vi "cblas zherk.vi"(0 "A":T4, 2 "C":T4, 3 "alpha":dbl=1.0, 4 "beta":dbl=1.0, 5 "order":T3=101 items=["CblasRowMajor"=101, "CblasColMajor"=102], 6 "transA":T1=111 items=["CblasNoTrans"=111, "CblasTrans"=112, "CblasConjTrans "=113], 7 "uplo":T2=121 items=["CblasUpper"=121, "CblasLower"=122], 8 "lda":i32, 11 "n":i32=-1, 12 "ldc":i32, 13 "k":i32=-1) -> (14 "zherk":T4, 19 "error":i32)   [LabVIEW 2017, in "NI_AALBLAS.lvlib"]
uses:
  NI_AALBLAS.lvlib
  ComplexMatrix.ctl
  Order.ctl
  UpLo.ctl
  Operation_Transpose.ctl
  NI_Matrix.lvlib
  lvblas.dll
panel:
  # "void cblas_zherk(order, uplo, transA, n, k, alpha,*A, lda, beta, *C, ldc)"
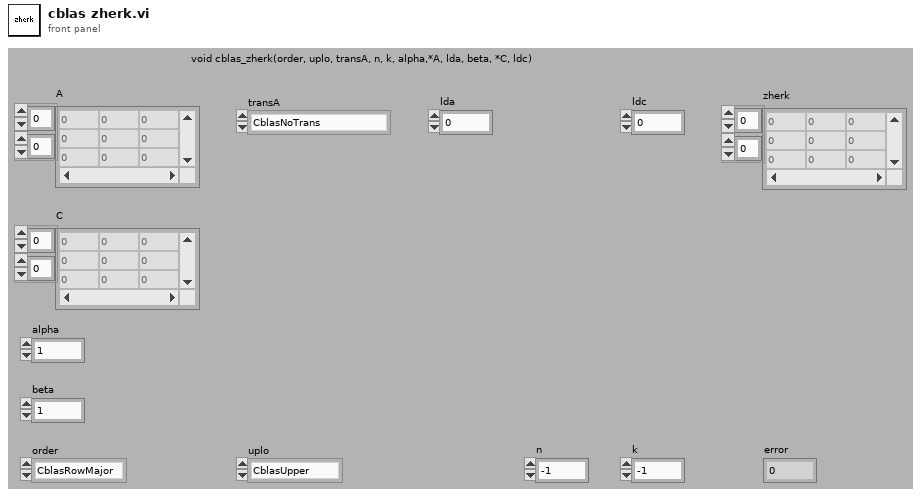
[diagram p1: front panel]
types:
  T1 = typedef "NI_AALBLAS.lvlib/Operation_Transpose.ctl" = i32
  T2 = typedef "NI_AALBLAS.lvlib/UpLo.ctl" = i32
  T3 = typedef "NI_AALBLAS.lvlib/Order.ctl" = i32
  T4 = typedef "NI_Matrix.lvlib/ComplexMatrix.ctl" = cdb[][]
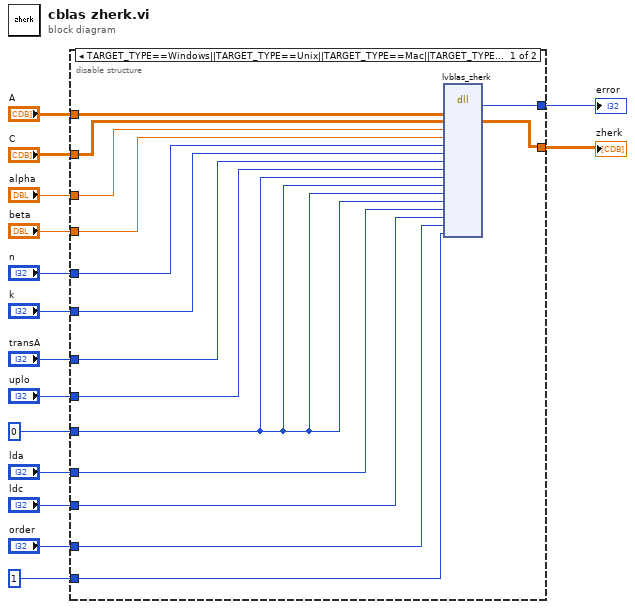
[diagram p0: block diagram]
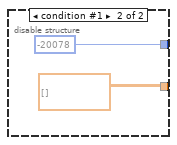
[diagram p2: hidden frame]
diagram:
  n1 = disable-structure shown="TARGET_TYPE==Windows||TARGET_TYPE==Unix||TARGET_TYPE==Mac||TARGET_TYPE==RT" {
    disable-tunnel: [w30 -20078 ("error")] -> w15
    disable-tunnel: "A" -> [w29 _]
    disable-tunnel: "C" -> [w28 _]
    disable-tunnel: "alpha" -> [w27 _]
    disable-tunnel: [w22 T4 [] ("Complex Matrix")] -> w14
    disable-tunnel: "uplo" -> [w25 _]
    disable-tunnel: 0 -> [w23 _]
    disable-tunnel: "beta" -> [w26 _]
    disable-tunnel: "transA" -> [w24 _]
    disable-tunnel: "order" -> [w21 _]
    disable-tunnel: "n" -> [w20 _]
    disable-tunnel: "k" -> [w19 _]
    disable-tunnel: "lda" -> [w18 _]
    disable-tunnel: "ldc" -> [w17 _]
    disable-tunnel: 1 -> [w16 _]
    frame condition #0 (active) {
      n2 = dll-call lib="C:/Program Files/National Instruments/LabVIEW 2017/resource/lvblas.*" fn="lvblas_zherk" ("CBLAS.dll:MtrxxMtrxH")("A"=w29, "C"=w28, "alpha"=w27, "beta"=w26, "n"=w20, "k"=w19, "trans"=w24, "uplo"=w25, "startARow"=w23, "startACol"=w23, "startCRow"=w23, "startCCol"=w23, "lda"=w18, "ldc"=w17, "order"=w21, "check"=w16) -> ("error"=w30:i32, "C"=w22:T4)  [unwired: 18 in, 2 out]
    }
    frame condition #1 {
    }
  }
  "zherk" <- w14
  "error" <- w15
